vi "Multichannel demo2015.vi"() -> ()   [LabVIEW 2015]
uses:
  Examples/Labview/V12/base_xml.llb/Type Descriptor Enumeration__ogtk.ctl
panel:
  out "size(s) 2":i32[](array[numeric])
  out "State":i32
  out "TechniqueID":i32
  out "Data1 3":dbl[][](array[numeric])
  out "Data1 2":dbl[][](array[numeric])
  out "Data1":dbl[][](array[numeric])
  out "Channel 1 exe":T1 {"NbAmp" min=5 max=7; "LcBoard" min=5 max=7; "AmpCode" min=5 max=7}
  out "Channel 2 exe":T1 {"NbAmp" min=5 max=7; "LcBoard" min=5 max=7; "AmpCode" min=5 max=7}
  out "Channel 3 exe":T1 {"NbAmp" min=5 max=7; "LcBoard" min=5 max=7; "AmpCode" min=5 max=7}
  out "Channel 3":T1 {"NbAmp" min=5 max=7; "LcBoard" min=5 max=7; "AmpCode" min=5 max=7}
  out "Channel  2":T1 {"NbAmp" min=5 max=7; "LcBoard" min=5 max=7; "AmpCode" min=5 max=7}
  out "Channel 1":T1 {"NbAmp" min=5 max=7; "LcBoard" min=5 max=7; "AmpCode" min=5 max=7}
  out "size(s)":i32=16
  out "Plugged channels 2":i32[](array[numeric])=[1, 0, 0, 0, 0, 0, 0, 0, 0, 0, 0, 0, 0, 0, 0, 0]
  out "error out":errorcluster
  out "Plugged channels":i32[](array[numeric])=[1, 0, 0, 0, 0, 0, 0, 0, 0, 0, 0, 0, 0, 0, 0, 0]
  in  "VSCAN Parameters":T2={"tb"=5e-05, "vs_initial "=TRUE, "Voltage_step"=0.0, "Scans"=[{" vs_initial "=FALSE, "Voltage_step"=0.1, "Scan_Rate"=0.1}, {" vs_initial "=FALSE, "Voltage_step"=-0.2, "Scan_Rate"=0.1}, {" vs_initial "=FALSE, "Voltage_step"=0.0, "Scan_Rate"=0.1}], "Scan_number"=2, "N_Cycles"=0, "Record_every_dE"=0.01, "Begin_measuring_I"=0.5, "End_measuring_I"=0.75, "I_Range"=12, "E_Range"=3, "Bandwidth"=5, "em"=1, "ce"=0} {"tb" min=5e-05 max=1 format="%^_3e"; "ce" items=["Standard", "CE to ground"]; "End_measuring_I" min=0 max=1 format="%.2f"; "Begin_measuring_I" min=0 max=1 format="%.2f"; "Voltage_step" min=-10 max=10 format="%^_3e"; "N_Cycles" min=0 max=1000000; "Scan_number" min=0 max=98; "Scans"."Scan_Rate" min=1e-05 max=10 format="%^_3e"; "Scans"."Voltage_step" format="%^_3e"; "E_Range" items=["±2.5V", "±5V", "±10V", "Auto"]; "Bandwidth" items=["1"=1, "2"=2, "3"=3, "4"=4, "5"=5, "6"=6, "7"=7, "8"=8, "9"=9]; "Record_every_dE" format="%^_3e"; "I_Range" items=["1pA", "1nA", "10nA", "100nA", "1µA", "10µA", "100µA", "1mA", "10mA", "100mA", "1A", "Booster", "Auto"]}
  out "BW disabled ranges":i32[](array[numeric])=[7, 8, 9, 10]
  out "current disabled ranges":i32[](array[numeric])=[0, 1, 2, 3, 4]
  out "Channel initial":T1={"Channel"=0, "BoardVersion"=13, "BoardSerialCode"=6878, "FirmwareCode"=5, "FirmwareVersion"=5280, "XilinxVersion"=42511, "AmpCode"=15, "NbAmp"=0, "LcBoard"=0, "Zboard"=1, "MuxBoard"=0, "GPRAboard"=0, "MemSize"=786432, "MemFilled"=0, "state"=0, "MaxIRange"=10, "MinIRange"=5, "MaxBandwidth"=7, "NbOfTechniques"=0} {"NbAmp" min=5 max=7; "LcBoard" min=5 max=7; "AmpCode" min=5 max=7}
  out "Number of available Channels":u32=16
  out "ID":i32=1
  in  "First Channels":u8(ring) items=["1", "2", "3", "4", "5", "6", "7", "8", "9", "10", "11", "12", "13", "14", "15", "16"]
  out "Device Code":i32=6
  out "TDeviceINfo":T3={"Device Code"=6, "RAM size"=32, "CPU"=9200, "Nb of channels"=1, "nb of slots"=5, "Firmware version"=1116, "Firmware date_Y"=2017, "Firmware date_M"=10, "Firmware date_D"=12, "HT displayON"=1, "Nb of connected PC"=1} {"nb of slots" min=5 max=7}
  in  "IP adress":string="USB0"
  # "Note: channel starts from 0 to 15"
  # "status 0= finished, 1=not finshed,"
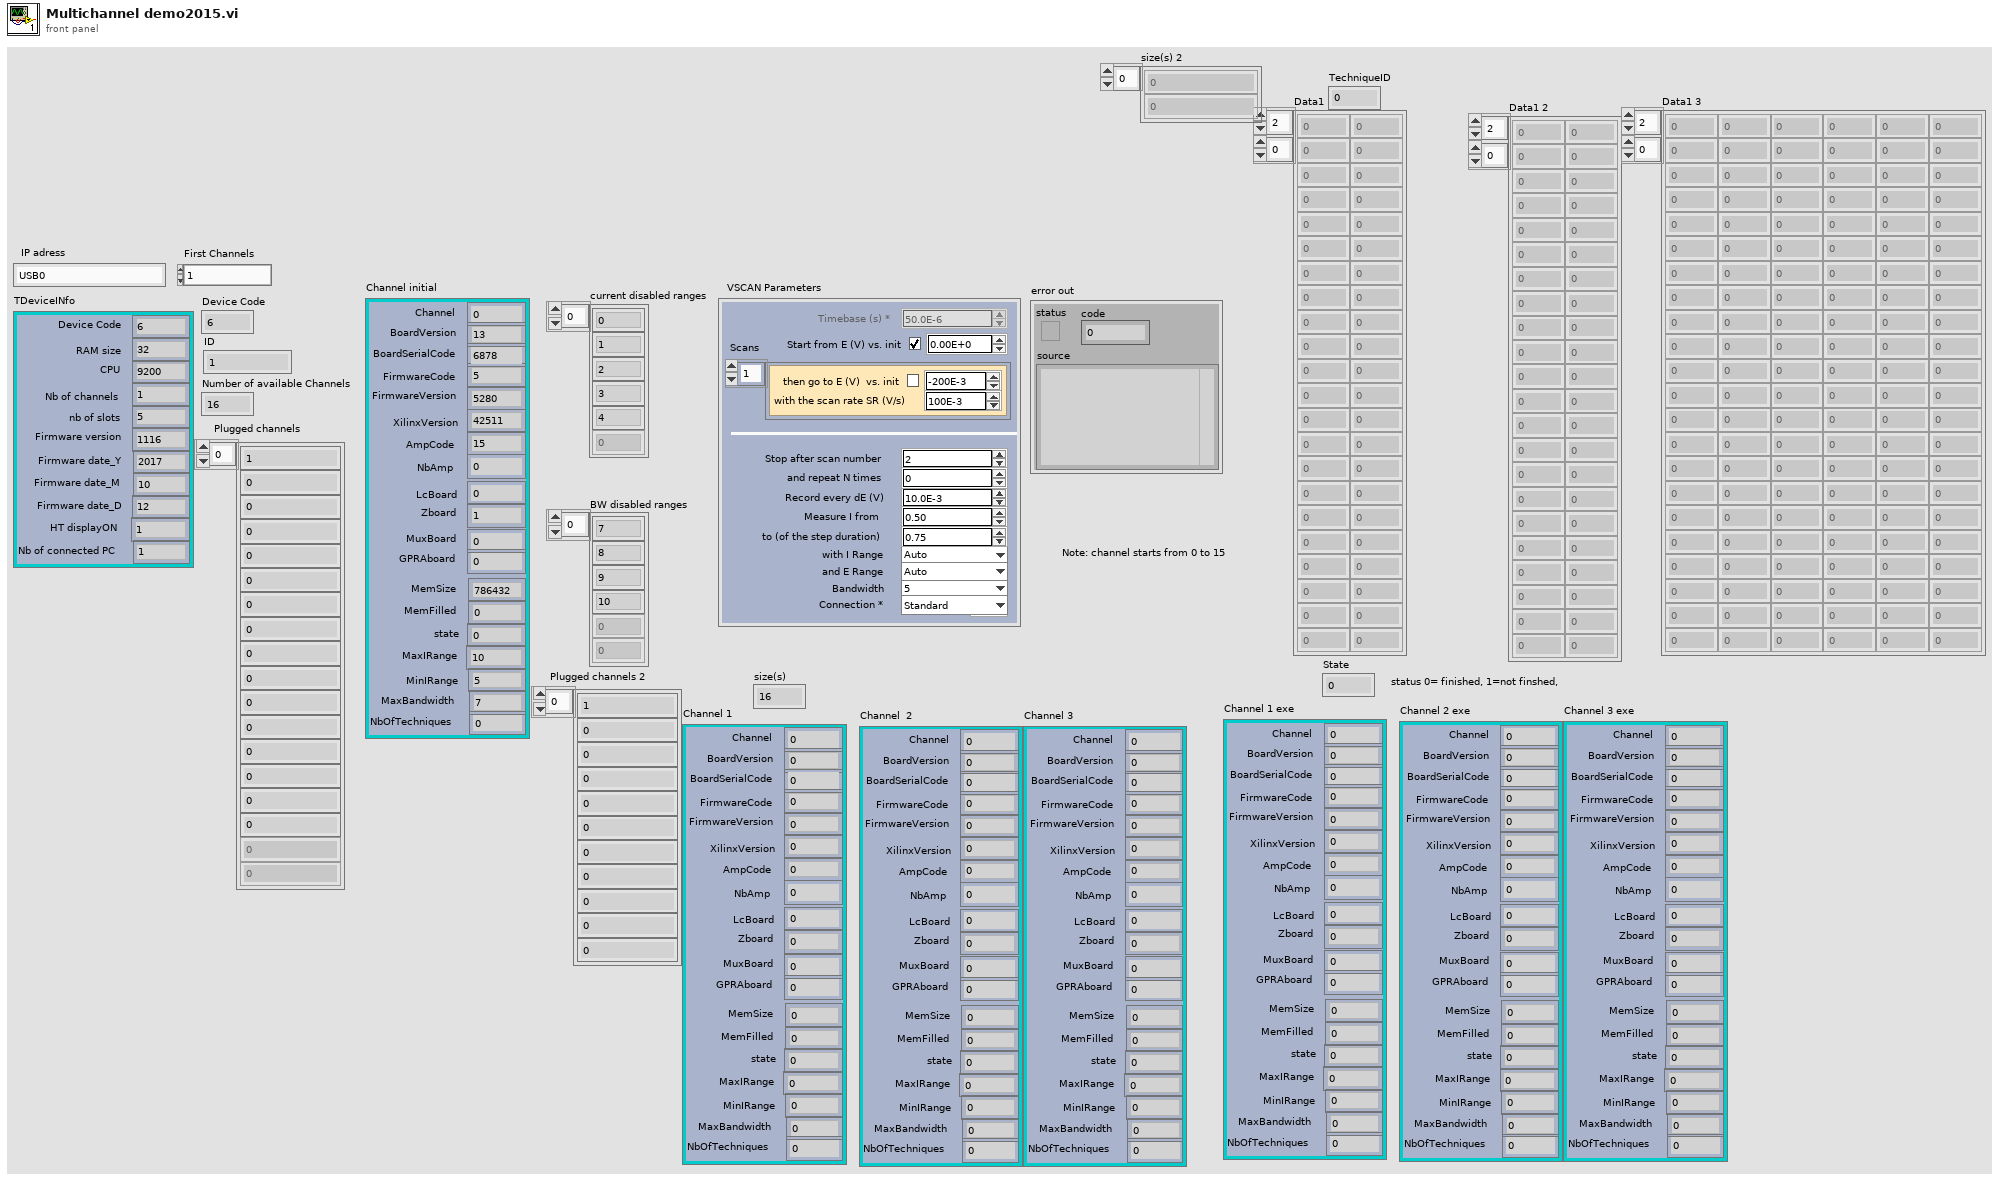
[diagram p1: front panel]
types:
  T1 = cluster{"Channel":i32, "BoardVersion":i32, "BoardSerialCode":i32, "FirmwareCode":i32, "FirmwareVersion":i32, "XilinxVersion":i32, "AmpCode":i32, "NbAmp":i32, "LcBoard":i32, "Zboard":i32, "MuxBoard":i32, "GPRAboard":i32, "MemSize":i32, "MemFilled":i32, "state":i32, "MaxIRange":i32, "MinIRange":i32, "MaxBandwidth":i32, "NbOfTechniques":i32}
  T2 = cluster{"tb":sgl, "vs_initial ":bool, "Voltage_step":sgl, "Scans":cluster{" vs_initial ":bool, "Voltage_step":sgl, "Scan_Rate":sgl}[], "Scan_number":i32, "N_Cycles":i32, "Record_every_dE":sgl, "Begin_measuring_I":sgl, "End_measuring_I":sgl, "I_Range":u16, "E_Range":u16, "Bandwidth":u16, "em":u16, "ce":u16}
  T3 = cluster{"Device Code":i32, "RAM size":i32, "CPU":i32, "Nb of channels":i32, "nb of slots":i32, "Firmware version":i32, "Firmware date_Y":i32, "Firmware date_M":i32, "Firmware date_D":i32, "HT displayON":i32, "Nb of connected PC":i32}
  T4 = typedef "Type Descriptor Enumeration__ogtk.ctl" = enum8{"<Null>", "I8", "I16", "I32", "I64", "U8", "U16", "U32", "U64", "SGL", "DBL", "EXT", "CSG", "CDB", "CXT", "0x0F", "0x10", "0x11", "0x12", "0x13", "0x14", "Enum U8", "Enum U16", "Enum U32", "Enum U64", "SGL PQ", "DBL PQ", "EXT PQ", "CSG PQ", "CDB PQ", "CXT PQ", "0x1F", "0x20", "Boolean", "0x22", "0x23", "0x24", "0x25", "0x26", "0x27", "0x28", "0x29", "0x2A", "0x2B", "0x2C", "0x2D", "0x2E", "0x2F", "String", "0x31", "Path", "Pict", "0x34", "0x35", "0x36", "DAQ", "0x38", "0x39", "0x3A", "0x3B", "0x3C", "0x3D", "0x3E", "0x3F", "Array", "0x41", "0x42", "0x43", "0x44", "0x45", "0x46", "0x47", "0x48", "0x49", "0x4A", "0x4B", "0x4C", "0x4D", "0x4E", "0x4F", "Cluster", "0x51", "0x52", "Variant", "Waveform", "0x55", "0x56", "0x57", "0x58", "0x59", "0x5A", "0x5B", "0x5C", "0x5D", "0x5E", "0x5F", "0x60", "0x61", "0x62", "0x63", "0x64", "0x65", "0x66", "0x67", "0x68", "0x69", "0x6A", "0x6B", "0x6C", "0x6D", "0x6E", "0x6F", "Refnum"}
  T5 = cluster{"Data Type":T4, "Format String":string}[]
  T6 = cluster{" vs_initial ":bool, "Voltage_step":sgl, "Scan_Rate":sgl}[]
  T7 = cluster{" vs_initial ":bool, "Voltage_step":sgl, "Scan_Rate":sgl}
  T8 = cluster{"Label":string, "type":i32, "valeur":u32, "index":i32}[]
  T9 = cluster{"IRQskipped":i32, "NbRaws":i32, "NbCols":i32, "Technique Index":i32, "TechniqueID":i32, "PrcessIndex":i32, "loop":i32, "StartTime":dbl, "MuxPad":i32}
  T10 = cluster{"State":i32, "MemFilled":i32, "TimeBase":sgl, " Ewe":sgl, " EweRangeMin":sgl, " EweRangeMax":sgl, "Ece":sgl, "EceRangeMin":sgl, "EceRangeMax":sgl, "Eoverflow":i32, "I":sgl, "IRange":i32, "Ioverflow":i32, "ElapsedTime":sgl, "Freq":sgl, "Rcomp":sgl, "Saturation":sgl, "OptErr":i32, "OptPos":i32}
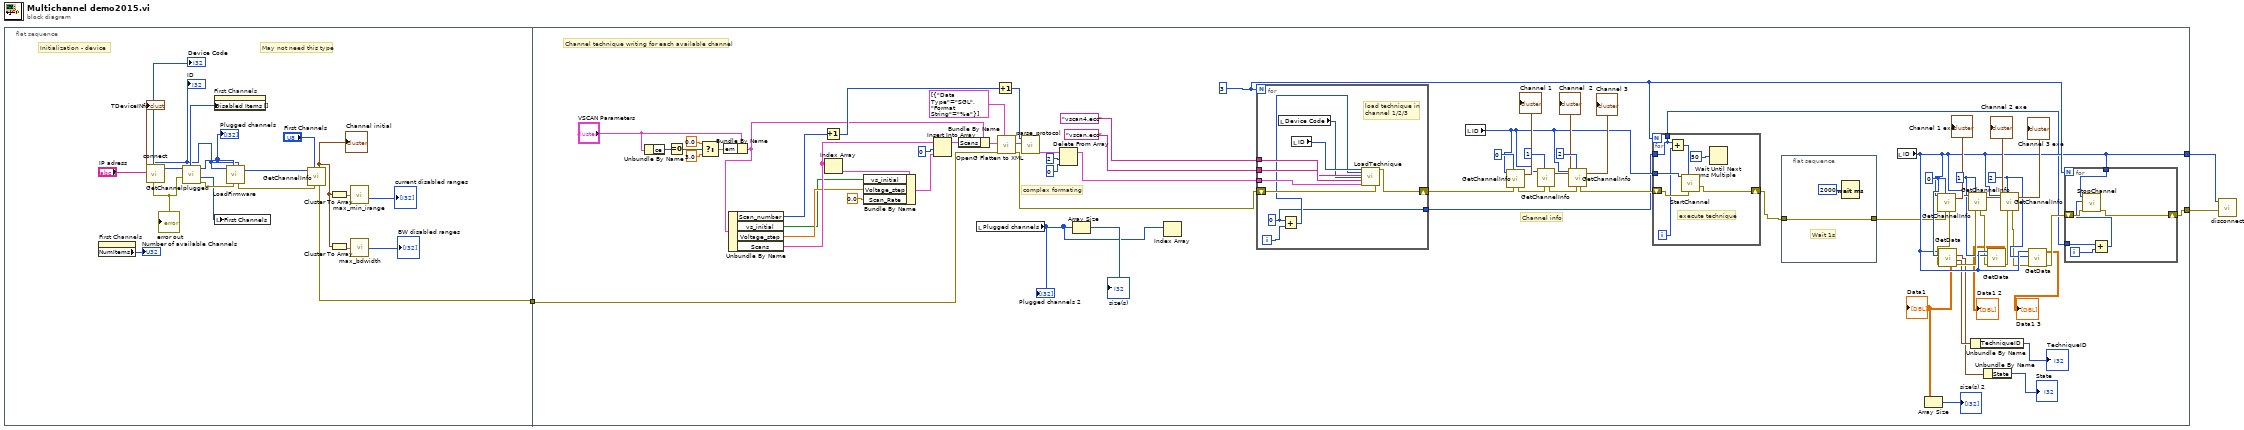
[diagram p0: block diagram]
diagram:
  n1 = flat-sequence {
    tunnel: [w4] -> w3
    tunnel: w3 -> [w61]
    tunnel: [w45] -> w2
    tunnel: [w40] -> w1
    frame #0 {
      # "May not need this type"
      # "Initialization - device"
      n2 = property on="First Channels" class="Ring (strict)"() -> ("NumItems"=→"Number of available Channels":u32)  [unwired: 2 in, 2 out]
      n3 = call "connect.vi"("IP"="IP adress") -> ("error out"=w19:errorcluster, "Device Code"=→"Device Code":i32, "TDeviceINfo"=→"TDeviceINfo":T3, "ID"=w9:i32)  [unwired: 7 in]
      "ID" <- w9
      "error out" <- w19
      n4 = call "GetChannelplugged.vi"("error in (no error)"=w19, "ID"=w9) -> ("error out"=w18:errorcluster, "First channel"=w10:i32, "Disabled channels"=w15:i32[], "Plugged channels"=w20:i32[])  [unwired: 6 in]
      "Plugged channels" <- w20
      n5 = property on="First Channels" class="Ring (strict)"("Disabled Items []"=w15) -> ()  [unwired: 2 in, 2 out]
      n6 = local write "First Channels"(w10) -> ()
      n7 = call "LoadFirmware.vi"("error in (no error)"=w18, "Channels"=w20, "ID"=w9) -> ("error out"=w8:errorcluster)  [unwired: 7 in, 1 out]
      n8 = call "GetChannelInfo.vi"("error in (no error)"=w8, "Channel"="First Channels", "ID"=w9) -> ("error out"=w4:errorcluster, "Channel information"=w11:T1)  [unwired: 7 in]
      "Channel initial" <- w11
      n9 = Cluster To Array(cluster=w11) -> (array=w13:i32[])
      n10 = Cluster To Array(cluster=w11) -> (array=w12:i32[])
      n11 = call "max_min_irange.vi"("resources"=w13) -> ("disabled ranges"=→"current disabled ranges":i32[])
      n12 = call "max_bdwidth.vi"("resources"=w12) -> ("disabled ranges"=→"BW disabled ranges":i32[])
    }
    frame #1 {
      w38 = u8 2 ("Channel")
      w39 = u8 1 ("Channel")
      w43 = u8 0 ("Channel")
      w44 = 3
      # "Channel info"
      # "complex formating"
      # "Channel technique writing for each available channel"
      n13 = Unbundle By Name("VSCAN Parameters") -> ("ce"=w69:u16)
      n14 = Equal To 0?(x=w69) -> (x = 0?=w68:bool)
      n15 = Select(t=0.0, s=w68, f=3.0) -> (s? t:f=w71:dbl)
      n16 = Bundle By Name(cluster="VSCAN Parameters", "em"=w71) -> (w65:T2)
      n17 = Unbundle By Name(w65) -> ("Scan_number"=w74:i32, "vs_initial"=w79:bool, "Voltage_step"=w80:sgl, "Scans"=w83:T6)
      n18 = Increment(x=w74) -> (x+1=w75:i32)
      n19 = Index Array(array=w83) -> (element=w77:T7)  [unwired: 1 in]
      n20 = Bundle By Name(cluster=w77, "vs_initial"=w79, "Voltage_step"=w80, "Scan_Rate"=sgl 0.0) -> (w81:T7)
      n21 = Insert Into Array(array=w83, index=0 ("indice"), new element=w81) -> (w84:T6)
      n22 = Bundle By Name(cluster=w65, "Scans"=w84) -> (w76:T2)
      n23 = local read "Plugged channels"() -> (w62:i32[])
      "Plugged channels 2" <- w62
      n24 = Increment(x=w75) -> (x+1=w73:i32)
      n25 = call "OpenG Flatten to XML.vi"("Type Formats (default)"=T5 [{"Data Type"=enum."SGL", "Format String"="%e"}] ("Type Formats"), "error in (no error)"=w61, "LabVIEW Data"=w76) -> ("error out"=w53:errorcluster, "XML String"=w88:string)  [unwired: 7 in]
      n26 = call "parse_protocol.vi"("XML String In"=w88, "index array"=w73) -> ("Params Values"=w85:T8)  [unwired: 7 in]
      n27 = Delete From Array(array=w85, length=2 ("longueur"), index=0 ("indice")) -> (array with subset deleted=w64:T8)  [unwired: 1 out]
      n28 = Array Size(array=w62) -> (size(s)=→"size(s)":i32)
      n29 = Index Array(array=w62) -> ()  [unwired: 1 in, 1 out]
      n30 = for {
        N: w44 -> [_]
        tunnel: "vscan.ecc" ("FName") -> [w115]
        tunnel: "vscan4.ecc" ("FName") -> [w114]
        tunnel: w64 -> [w113]
        shift-right: [w110] -> w54
        shift-left: w53 -> [w109]
        tunnel: [w106] -> w23
        i -> [w108]
        w106 = 0 ("x")
        # "load technique in\nchannel 1/2/3"
        n31 = local read "Device Code"() -> (w111:i32)
        n32 = Add(x=w106, y=w108) -> (x+y=w107:i32)
        n33 = local read "ID"() -> (w112:i32)
        n34 = call "LoadTechnique.vi"("ID"=w112, "Selected Channel"=w107, "FName4"=w114, "Device Code"=w111, "FName"=w115, "Protocol Parameters"=w113, "error in (no error)"=w109) -> ("error out"=w110:errorcluster)  [unwired: 12 in]
      }
      n35 = local read "ID"() -> (w50:i32)
      n36 = call "GetChannelInfo.vi"("error in (no error)"=w54, "Channel"=u8 0, "ID"=w50) -> ("error out"=w52:errorcluster, "Channel information"=→"Channel 1":T1)  [unwired: 7 in]
      n37 = call "GetChannelInfo.vi"("error in (no error)"=w52, "Channel"=u8 1, "ID"=w50) -> ("error out"=w51:errorcluster, "Channel information"=→"Channel  2":T1)  [unwired: 7 in]
      n38 = call "GetChannelInfo.vi"("error in (no error)"=w51, "Channel"=u8 2, "ID"=w50) -> ("error out"=w49:errorcluster, "Channel information"=→"Channel 3":T1)  [unwired: 7 in]
      n39 = for {
        N: w44 -> [_]
        tunnel: w50 -> [w105]
        shift-right: [w103] -> w31
        shift-left: w49 -> [w104]
        tunnel: w23 -> [w99]
        tunnel: [w99] -> w22
        i -> [w100]
        # "execute technique"
        n40 = Add(x=w99, y=w100) -> (x+y=w101:i32)
        n41 = call "StartChannel.vi"("error in (no error)"=w104, "Channel"=w101, "ID"=w105) -> ("error out"=w103:errorcluster)  [unwired: 8 in]
        n42 = Wait Until Next ms Multiple(millisecond multiple=u32 50) -> ()  [unwired: 1 out]
      }
      n43 = flat-sequence {
        tunnel: w31 -> [w92]
        tunnel: [w92] -> w30
        frame #0 {
          # "Wait 1s"
          n44 = Wait (ms)(milliseconds to wait=u32 2000) -> ()  [unwired: 1 out]
        }
      }
      n45 = local read "ID"() -> (w40:i32)
      n46 = call "GetChannelInfo.vi"("error in (no error)"=w30, "Channel"=w43, "ID"=w40) -> ("error out"=w42:errorcluster, "Channel information"=→"Channel 1 exe":T1)  [unwired: 7 in]
      n47 = call "GetData.vi"("error in (no error)"=w42, "Channel"=w43, "ID"=w40) -> ("error out"=w41:errorcluster, "Data information"=w29:T9, "Current values"=w27:T10, "Data"=w25:dbl[][])  [unwired: 5 in]
      "Data1" <- w25
      n48 = Array Size(array=w25) -> (size(s)=→"size(s) 2":i32[])
      n49 = call "GetChannelInfo.vi"("error in (no error)"=w41, "Channel"=w39, "ID"=w40) -> ("error out"=w37:errorcluster, "Channel information"=→"Channel 2 exe":T1)  [unwired: 7 in]
      n50 = Unbundle By Name(w29) -> ("TechniqueID"=→"TechniqueID":i32)
      n51 = Unbundle By Name(w27) -> ("State"=→"State":i32)
      n52 = call "GetData.vi"("error in (no error)"=w37, "Channel"=w39, "ID"=w40) -> ("error out"=w36:errorcluster, "Data"=→"Data1 2":dbl[][])  [unwired: 5 in, 2 out]
      n53 = call "GetChannelInfo.vi"("error in (no error)"=w36, "Channel"=w38, "ID"=w40) -> ("error out"=w35:errorcluster, "Channel information"=→"Channel 3 exe":T1)  [unwired: 7 in]
      n54 = call "GetData.vi"("error in (no error)"=w35, "Channel"=w38, "ID"=w40) -> ("error out"=w34:errorcluster, "Data"=→"Data1 3":dbl[][])  [unwired: 5 in, 2 out]
      n55 = for {
        N: w44 -> [_]
        tunnel: w40 -> [w98]
        shift-right: [w96] -> w45
        shift-left: w34 -> [w97]
        tunnel: w22 -> [w93]
        i -> [w95]
        n56 = Add(x=w93, y=w95) -> (x+y=w94:i32)
        n57 = call "StopChannel.vi"("error in (no error)"=w97, "Channel"=w94, "ID"=w98) -> ("error out"=w96:errorcluster)  [unwired: 8 in]
      }
    }
  }
  n58 = call "disconnect.vi"("error in (no error)"=w2, "ID"=w1) -> ()  [unwired: 9 in, 1 out]
